vi "XY Graph Special Event Handler Core.vi"(8 "error in (no error)":errorcluster, 11 "XY Graph Event":T2) -> (0 "error out":errorcluster, 1 "Data":variant, 2 "Message":string, 3 "Menu Item Tag (dup)":string, 4 "Message Type":T1, 5 "Top Menu":string)   [LabVIEW 2021, in "XY Graph Add-Ons.lvlib"]
uses:
  XY Graph Add-Ons.lvlib
  XY Graph Event.ctl
  <vilib>/Utility/miscctls.llb/LVPoint32TypeDef.ctl
  Fits/Fit Plot Request Information.ctl
  <vilib>/Utility/miscctls.llb/LVPointDoubleTypeDef.ctl
  Fits/Fit Models.ctl
  XY Graph Mouse Click Event Data.ctl
  XY Graph Refnum.ctl
  XY Graph Save Plot Data.ctl
  Fits/Fits.lvlib
  Plot Editor/Plot Editor.lvlib
  Graphs.lvlib
  Histograms/Histogram Window.lvlib
  Strings/Strings.lvlib
  Rich Text Box/Text Format List.ctl
  Notebook/Notebook.lvlib
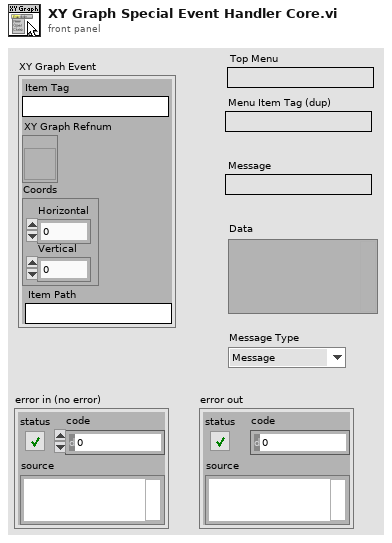
[diagram p1: front panel]
types:
  T1 = typedef "Notebook.lvlib/Text Format List.ctl" = enum16{"Message", "Result", "Error", "Setting", "Verbose", "Warning"}
  T2 = typedef "XY Graph Add-Ons.lvlib/XY Graph Event.ctl" = cluster{"Item Tag":string, "XY Graph Refnum":refnum<vi>, "Coords":T3, "Item Path":string}
  T3 = typedef "LVPoint32TypeDef.ctl" = cluster{"Horizontal":i32, "Vertical":i32}
  T4 = typedef "XY Graph Add-Ons.lvlib/XY Graph Mouse Click Event Data.ctl" = cluster{"Multiplot XY Graph":T5, "Mouse Coordinates":T3}
  T5 = typedef "XY Graph Add-Ons.lvlib/XY Graph Refnum.ctl" = refnum<vi>
  T6 = typedef "Fits.lvlib/Fit Plot Request Information.ctl" = cluster{"XY Graph Ref":refnum<vi>, "Mouse Coordinates":T7, "Fit Model":T8, "Plot Index":i32}
  T7 = typedef "LVPointDoubleTypeDef.ctl" = cluster{"X":dbl, "Y":dbl}
  T8 = typedef "Fits.lvlib/Fit Models.ctl" = enum16{"Select a Fit Model...", "           Single Peak", "Gaussian", "Asymmetric Gaussian", "Lorentzian", "Asymmetric Lorentzian", "Gaussian/Lorentzian", "Lorentzian/Gaussian", "           Double Peak", "Two Gaussians", "Two Asymmetric Gaussians", "Two H-Connected Gaussians", "Two T-Connected Gaussians", "Two H-Connected Asymmetric Gaussians", "Two T-Connected Asymmetric Gaussians", "           Triple Peak", "Three Gaussians", "Three Asymmetric Gaussians", "              Decays", "1-Exponential", "IRF*PSED", "2-Exponentials", "            Power Law", "Power Law", "Power Law with Offset", "               ACF", "2D Gaussian ACF", "2D Gaussian + Blinking ACF", "2D Gaussian + Flow ACF", "3D Gaussian ACF", "3D Gaussian + Blinking ACF", "             Multiplot", "2D Gaussian ACF & 2D Gaussian + Flow ACF"}
  T9 = typedef "XY Graph Add-Ons.lvlib/XY Graph Save Plot Data.ctl" = cluster{"XY Graph Refnum":refnum<vi>, "Mouse Coords":T3, "File Path":path}
  T10 = typedef "Graphs.lvlib/Plot Style 3.ctl" = cluster{"Plot Style":enum16{"unchanged", "Line", "Symbol", "Line + Symbol", "Histogram", "Histogram + Symbol"}, "Histogram Type":enum16{"unchanged", "Left Bound", "Center", "Right Bound"}, "Line Tickness":enum16{"unchanged", "Thin", "1 pixel", "2 pixel", "3 pixel", "4 pixel", "5 pixel"}, "Line Style":enum16{"unchanged", "Plain", "Long Dash", "Short Dash", "Long-Short Dash", "Long-Short-Short Dash"}, "Point Style":enum16{"unchanged", "None", "Empty Circle", "Filled Circle", "Thick Circle", "Dotted Circle", "Empty Square", "Filled Square", "Thick Square", "Dotted Square", "Small Filled Square", "Dot", "Cross", "Tiny Cross", "Large X", "Small x", "Diamond", "Small Empty Square"}, "Line Color":u32, "Point Color":u32, "Anti-aliased":bool, "Line Color Chooser":enum16{"unchanged", "Color Box", "Color List"}, "Point Color Chooser":enum16{"unchanged", "Color Box", "Color List"}, "Line Color List":string, "Point Color List":string}
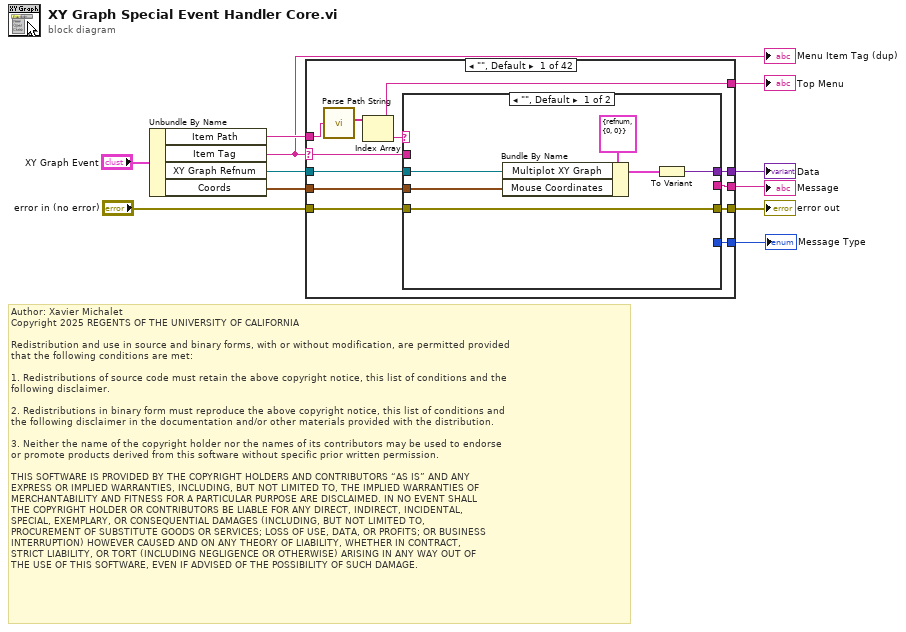
[diagram p0: block diagram]
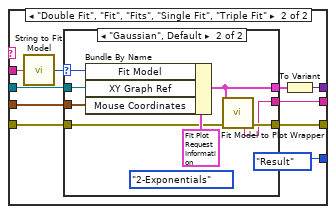
[diagram p2: hidden frame]
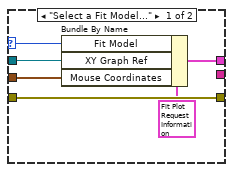
[diagram p3: hidden frame]
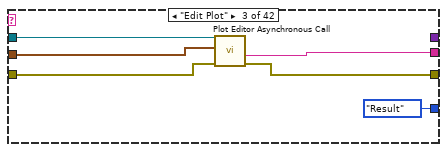
[diagram p5: hidden frame]
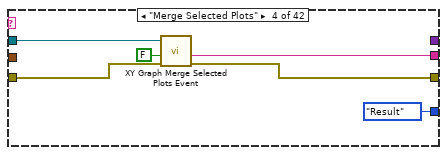
[diagram p6: hidden frame]
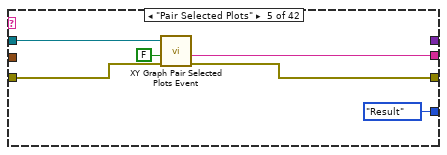
[diagram p7: hidden frame]
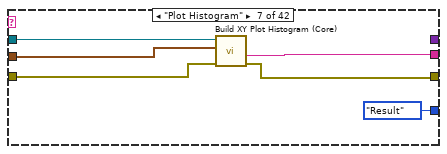
[diagram p9: hidden frame]
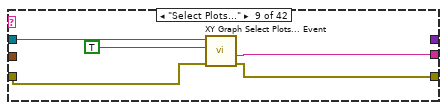
[diagram p11: hidden frame]
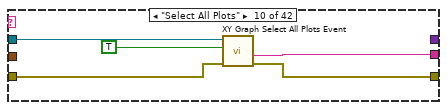
[diagram p12: hidden frame]
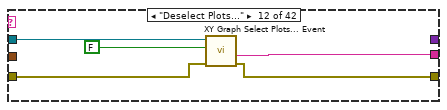
[diagram p14: hidden frame]
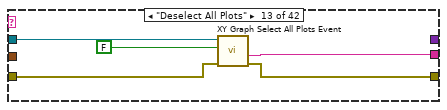
[diagram p15: hidden frame]
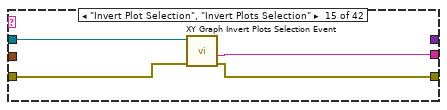
[diagram p17: hidden frame]
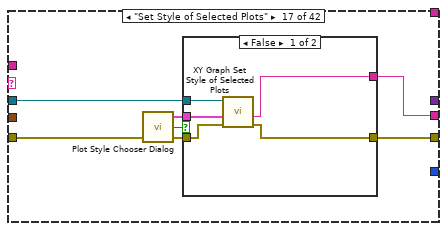
[diagram p19: hidden frame]
diagram:
  # "Author: Xavier Michalet\nCopyright 2025 REGENTS OF THE UNIVERSITY OF CALIFORNIA\n\nRedistribution and use in source and binary forms, with or without modification, are permitted provided\nthat the following conditions are met:\n\n1. Redistributions of source code must retain the above copyright notice, this list of conditions and the\nfollowing disclaimer.\n\n2. Redistributions in binary form must reproduce the above copyright notice, this list of conditions and\nthe following disclaimer in the documentation and/or other materials provided with the distribution.\n\n3. Neither the name of the copyright holder nor the names of its contributors may be used to endorse \nor promote products derived from this software without specific prior written permission.\n\nTHIS SOFTWARE IS PROVIDED BY THE COPYRIGHT HOLDERS AND CONTRIBUTORS “AS IS” AND ANY \nEXPRESS OR IMPLIED WARRANTIES, INCLUDING, BUT NOT LIMITED TO, THE IMPLIED WARRANTIES OF\nMERCHANTABILITY AND FITNESS FOR A PARTICULAR PURPOSE ARE DISCLAIMED. IN NO EVENT SHALL\nTHE COPYRIGHT HOLDER OR CONTRIBUTORS BE LIABLE FOR ANY DIRECT, INDIRECT, INCIDENTAL, \nSPECIAL, EXEMPLARY, OR CONSEQUENTIAL DAMAGES (INCLUDING, BUT NOT LIMITED TO, \nPROCUREMENT OF SUBSTITUTE GOODS OR SERVICES; LOSS OF USE, DATA, OR PROFITS; OR BUSINESS\nINTERRUPTION) HOWEVER CAUSED AND ON ANY THEORY OF LIABILITY, WHETHER IN CONTRACT, \nSTRICT LIABILITY, OR TORT (INCLUDING NEGLIGENCE OR OTHERWISE) ARISING IN ANY WAY OUT OF\nTHE USE OF THIS SOFTWARE, EVEN IF ADVISED OF THE POSSIBILITY OF SUCH DAMAGE."
  n1 = Unbundle By Name("XY Graph Event") -> ("Item Path"=w6:string, "Item Tag"=w5:string, "XY Graph Refnum"=w4:refnum<vi>, "Coords"=w3:T3)
  "Menu Item Tag (dup)" <- w5
  n2 = case shown="\"\", Default" w5 {
    selector: w5 -> [w20 _ _ _ _ _ _ _ _ _ _ _ _ _ _ _ _ _ _ _ _ _ _ _ _ _ _ _ _ _ _ _ _ _ _ _ _ _ _ _ _ _]
    tunnel: w4 -> [w22 _ w59 w65 w71 _ w78 _ w84 w89 _ w95 w100 _ w105 _ w110 w121 _ w131 w137 w141 _ w144 w153 w158 _ w167 w172 _ w180 _ w188 w194 _ w203 w211 w219 w224 _ w229 w233]
    tunnel: w3 -> [w21 _ w58 _ _ _ w77 _ _ _ _ _ _ _ _ _ _ _ _ w130 _ _ _ w143 _ _ _ _ _ _ w179 _ _ _ _ w202 w210 w218 _ _ _ _]
    tunnel: "error in (no error)" -> [w17 w53 w57 w63 w69 w72 w76 w79 w83 w87 w90 w94 w98 w101 w104 w106 w109 w123 w124 w129 w136 w140 w142 w149 w154 w159 w160 w166 w171 w173 w177 w182 w185 w191 w195 w200 w208 w216 w223 w225 w228 w232]
    tunnel: [w16 w53 w56 w62 w68 w72 w75 w79 w81 w85 w90 w92 w96 w101 w103 w106 w108 w122 w124 w127 w135 w139 w142 w148 w152 w157 w160 w165 w168 w173 w176 w182 w186 w192 w195 w199 w207 w215 w222 w225 w227 w231] -> w10
    tunnel: [w15 _ w55 w61 w67 _ w74 _ w80 w86 _ w91 w97 _ w102 _ w107 w120 _ w128 w134 w138 _ w147 w150 w155 _ w164 w170 _ w175 _ w184 w190 _ w198 w206 w214 w221 _ w226 w230] -> w11
    tunnel: w6 -> [w19 _ _ _ _ _ _ _ _ _ _ _ _ _ _ _ _ _ _ _ _ _ _ _ _ _ _ _ _ _ _ _ _ _ _ _ _ _ _ _ _ _]
    tunnel: [w14 _ _ _ _ _ _ _ _ _ _ _ _ _ _ _ _ _ _ w125 w132 _ _ _ _ _ _ w163 w169 _ _ _ _ _ _ _ _ _ _ _ _ _] -> w8
    tunnel: [w13 _ _ _ _ _ _ _ _ _ _ _ _ _ _ _ _ _ _ _ _ _ _ _ _ _ _ _ _ _ _ _ _ _ _ _ _ _ _ _ _ _] -> w2
    tunnel: [w12 _ Text_Format_List."Result" ("Message Type") Text_Format_List."Result" ("Message Type") Text_Format_List."Result" ("Message Type") _ Text_Format_List."Result" ("Message Type") _ _ _ _ _ _ _ _ _ _ _ _ _ _ _ _ _ _ _ _ _ _ _ Text_Format_List."Result" ("Message Type") _ Text_Format_List."Result" ("Message Type") Text_Format_List."Result" ("Message Type") _ Text_Format_List."Result" ("Message Type") Text_Format_List."Result" ("Message Type") Text_Format_List."Result" ("Message Type") Text_Format_List."Result" ("Message Type") _ _ _] -> w1
    frame "", Default {
      (unwired) T6 {"XY Graph Ref"=refnum, "Mouse Coordinates"={"X"=0.0, "Y"=0.0}, "Fit Model"=enum."Select a Fit Model...", "Plot Index"=-1} ("output cluster")
      n3 = call "Parse Path String.vi"("Path in"=w19) -> ("Folder Hierarchy"=w18:string[])  [unwired: 4 in, 1 out]
      n4 = Index Array(array=w18) -> (element=w13:string)  [unwired: 1 in]
      n5 = case shown="\"\", Default" w13 {
        tunnel: w22 -> [w26 w38]
        tunnel: w21 -> [w25 w37]
        tunnel: w20 -> [_ w36]
        tunnel: w17 -> [w28 w34]
        tunnel: [w28 w33] -> w16
        tunnel: [_ w32] -> w15
        tunnel: [w23 w30] -> w14
        tunnel: [_ Text_Format_List."Result" ("Message Type")] -> w12
        frame "", Default {
          n6 = Bundle By Name(cluster=T4 {"Multiplot XY Graph"=refnum, "Mouse Coordinates"={"Horizontal"=0, "Vertical"=0}} ("Mouse Click Event Data"), "Multiplot XY Graph"=w26, "Mouse Coordinates"=w25) -> (w24:T4)
          n7 = To Variant(anything=w24) -> (Variant=w23:variant)
        }
        frame "Double Fit", "Fit", "Fits", "Single Fit", "Triple Fit" {
          n8 = call "String to Fit Model.vi"("String"=w36) -> ("Fit Model"=w35:T8)  [unwired: 8 in]
          n9 = case shown="\"Gaussian\", Default" w35 {
            selector: w35 -> [w43 w49]
            tunnel: w38 -> [w42 w50]
            tunnel: w37 -> [w41 w51]
            tunnel: w34 -> [w44 w48]
            tunnel: [w44 w47] -> w33
            tunnel: [_ w46] -> w32
            tunnel: [w39 w45] -> w31
            frame "Select a Fit Model..." {
              n10 = Bundle By Name(cluster=T6 {"XY Graph Ref"=refnum, "Mouse Coordinates"={"X"=0.0, "Y"=0.0}, "Fit Model"=enum."Select a Fit Model...", "Plot Index"=0} ("Fit Plot Info"), "Fit Model"=w43, "XY Graph Ref"=w42, "Mouse Coordinates"=w41) -> (w39:T6)
            }
            frame "Gaussian", Default {
              (unwired) Fit_Models."2-Exponentials" ("Fit Model")
              n11 = Bundle By Name(cluster=T6 {"XY Graph Ref"=refnum, "Mouse Coordinates"={"X"=0.0, "Y"=0.0}, "Fit Model"=enum."Select a Fit Model...", "Plot Index"=-1} ("output cluster"), "Fit Model"=w49, "XY Graph Ref"=w50, "Mouse Coordinates"=w51) -> (w45:T6)
              n12 = call "Fit Model to Plot Wrapper.vi"("Fit Plot Info"=w45, "error in (no error)"=w48) -> ("Fit Result String"=w46:string, "error out"=w47:errorcluster)  [unwired: 5 in, 7 out]
            }
          }
          n13 = To Variant(anything=w31) -> (Variant=w30:variant)
        }
      }
    }
    frame "---------" {
    }
    frame "Edit Plot" {
      n14 = call "Plot Editor Asynchronous Call.vi"("error in (no error)"=w57, "Coords"=w58, "XYGraph in"=w59) -> ("Error Out"=w56:errorcluster, "Message"=w55:string)  [unwired: 5 in, 2 out]
    }
    frame "Merge Selected Plots" {
      n15 = call "XY Graph Merge Selected Plots Event.vi"("Error In"=w63, "Merge All Plots? (T)"=FALSE, "XY Graph Refnum"=w65) -> ("Error Out"=w62:errorcluster, "Message"=w61:string)  [unwired: 7 in]
    }
    frame "Pair Selected Plots" {
      n16 = call "XY Graph Pair Selected Plots Event.vi"("Error In"=w69, "Transpose?"=FALSE ("Merge All Plots? (T)"), "XYGraph Ref"=w71) -> ("Error Out"=w68:errorcluster, "Message"=w67:string)  [unwired: 7 in]
    }
    frame "-------------" {
    }
    frame "Plot Histogram" {
      n17 = call "Build XY Plot Histogram (Core).vi"("error in (no error)"=w76, "Mouse Click Coords (default: use Plot Index)"=w77, "XY Graph"=w78) -> ("error out"=w75:errorcluster, "Message"=w74:string)  [unwired: 6 in, 1 out]
    }
    frame "----------------" {
    }
    frame "Select Plots..." {
      n18 = call "XY Graph Select Plots... Event.vi"("Error In"=w83, "Select (T)/Deselect"=TRUE, "XYGraph Ref"=w84) -> ("Error Out"=w81:errorcluster, "Message"=w80:string)  [unwired: 4 in, 3 out]
    }
    frame "Select All Plots" {
      n19 = call "XY Graph Select All Plots Event.vi"("Error In"=w87, "Select (T)/Deselect"=TRUE, "XYGraph Ref"=w89) -> ("Error Out"=w85:errorcluster, "Message"=w86:string)  [unwired: 5 in, 2 out]
    }
    frame "----------------------" {
    }
    frame "Deselect Plots..." {
      n20 = call "XY Graph Select Plots... Event.vi"("Error In"=w94, "Select (T)/Deselect"=FALSE, "XYGraph Ref"=w95) -> ("Error Out"=w92:errorcluster, "Message"=w91:string)  [unwired: 4 in, 3 out]
    }
    frame "Deselect All Plots" {
      n21 = call "XY Graph Select All Plots Event.vi"("Error In"=w98, "Select (T)/Deselect"=FALSE, "XYGraph Ref"=w100) -> ("Error Out"=w96:errorcluster, "Message"=w97:string)  [unwired: 5 in, 2 out]
    }
    frame "-----------------------" {
    }
    frame "Invert Plot Selection", "Invert Plots Selection" {
      n22 = call "XY Graph Invert Plots Selection Event.vi"("Error In"=w104, "XYGraph Ref"=w105) -> ("Error Out"=w103:errorcluster, "Message"=w102:string)  [unwired: 6 in, 2 out]
    }
    frame "---------------" {
    }
    frame "Set Style of Selected Plots" {
      n23 = call "Plot Style Chooser Dialog.vi"("Error In"=w109) -> ("Plot Style out"=w113:T10, "Cancelled?"=w112:bool, "Error Out"=w111:errorcluster)  [unwired: 6 in]
      n24 = case shown="False" w112 {
        tunnel: w110 -> [w118 _]
        tunnel: w113 -> [w117 _]
        tunnel: w111 -> [w116 w119]
        tunnel: [w115 w119] -> w108
        tunnel: [w114 _] -> w107
        frame False {
          n25 = call "XY Graph Set Style of Selected Plots.vi"("Error In"=w116, "Plot Style"=w117, "XYGraph Ref"=w118) -> ("Error Out"=w115:errorcluster, "Message"=w114:string)  [unwired: 5 in, 2 out]
        }
        frame True {
        }
      }
    }
    frame "Set Axes of Selected Plots" {
      n26 = call "XY Graph Graph Axes Chooser Dialog.vi"("Error In"=w123, "XYGraph Ref"=w121) -> ("Error Out"=w122:errorcluster, "Message"=w120:string)  [unwired: 6 in, 2 out]
    }
    frame "-----------------" {
    }
    frame "Delete Plot" {
      n27 = call "XY Graph Delete Plot Event.vi"("Error In"=w129, "Mouse Click Coordinates"=w130, "XYGraph Ref"=w131) -> ("Error Out"=w127:errorcluster, "Message"=w128:string, "Deleted Plot Index"=w126:i32)  [unwired: 4 in, 2 out]
      n28 = To Variant(anything=w126) -> (Variant=w125:variant)
    }
    frame "Delete Selected Plots" {
      n29 = call "XY Graph Delete Selected Plots Event.vi"("Error In"=w136, "XYGraph Ref"=w137) -> ("Error Out"=w135:errorcluster, "Message"=w134:string, "Deleted Plot Indices"=w133:i32[])  [unwired: 5 in, 2 out]
      n30 = To Variant(anything=w133) -> (Variant=w132:variant)
    }
    frame "Clear Graph", "Delete All Plots" {
      n31 = call "XY Graph Clear Event.vi"("Error In"=w140, "XYGraph Ref"=w141) -> ("Error Out"=w139:errorcluster, "Message"=w138:string)  [unwired: 7 in, 1 out]
    }
    frame "------------------" {
    }
    frame "Save Plot" {
      n32 = Bundle By Name(cluster=T9 {"XY Graph Refnum"=refnum, "Mouse Coords"={"Horizontal"=0, "Vertical"=0}, "File Path"=path ""} ("AliGator Save Plot Data"), "XY Graph Refnum"=w144, "Mouse Coords"=w143) -> (w145:T9)
      n33 = call "XY Graph Save Plot Event.vi"("Error In"=w149, "AliGator Save Plot Data"=w145) -> ("Error Out"=w148:errorcluster, "Message"=w147:string)  [unwired: 4 in, 4 out]
    }
    frame "Save Selected Plots" {
      n34 = call "XY Graph Save Selected Plots Event.vi"("Error In"=w154, "Save All Plots? (T)"=FALSE, "XYGraph Ref"=w153) -> ("Error Out"=w152:errorcluster, "Message"=w150:string)  [unwired: 3 in, 4 out]
    }
    frame "Save All Plots" {
      n35 = call "XY Graph Save Selected Plots Event.vi"("Error In"=w159, "Save All Plots? (T)"=TRUE, "XYGraph Ref"=w158) -> ("Error Out"=w157:errorcluster, "Message"=w155:string)  [unwired: 3 in, 4 out]
    }
    frame "------------" {
    }
    frame "Load Plot(s)" {
      n36 = call "XY Graph Load Plot(s) Event.vi"("Error In"=w166, "XYGraph Ref"=w167) -> ("Error Out"=w165:errorcluster, "Message"=w164:string, "# Plots Added"=w162:i32[])  [unwired: 4 in, 3 out]
      n37 = Add Array Elements(numeric array=w162) -> (sum=w161:i32)
      n38 = To Variant(anything=w161) -> (Variant=w163:variant)
    }
    frame "Paste Plot(s) from Clipboard" {
      n39 = call "XY Graph Copy Plot(s) from Clipboard.vi"("error in (no error)"=w171, "XYGraph Ref"=w172) -> ("error out"=w168:errorcluster, "Message"=w170:string, "Number of Plots Added"=w169:i32)  [unwired: 7 in]
    }
    frame "--------------------------" {
    }
    frame "Transpose Plot" {
      n40 = Bundle(cluster=T4 {"Multiplot XY Graph"=refnum, "Mouse Coordinates"={"Horizontal"=0, "Vertical"=0}} ("Mouse Click Event Data"), "Multiplot XY Graph"=w180, "Mouse Coordinates"=w179) -> (w178:T4)
      n41 = call "XY Graph Transpose Plot Event.vi"("Error In"=w177, "Mouse Click Event Data"=w178) -> ("Error Out"=w176:errorcluster, "Message"=w175:string)  [unwired: 6 in, 2 out]
    }
    frame "--------------------" {
    }
    frame "Add Selected Plots" {
      n42 = call "XY Graph Sum Selected Plots Event.vi"("Error In"=w185, "Add All Plots? (F)"=FALSE, "XYGraph Ref"=w188) -> ("Error Out"=w186:errorcluster, "Message"=w184:string)  [unwired: 3 in, 4 out]
    }
    frame "Add All Plots" {
      n43 = call "XY Graph Sum Selected Plots Event.vi"("Error In"=w191, "Add All Plots? (F)"=TRUE, "XYGraph Ref"=w194) -> ("Error Out"=w192:errorcluster, "Message"=w190:string)  [unwired: 3 in, 4 out]
    }
    frame "---------------------" {
    }
    frame "Plot Arithmetic", "Single Plot Arithmetic", "y -> f(y) Transform", "y >> f(y) Transform" {
      n44 = Bundle(cluster=T4 {"Multiplot XY Graph"=refnum, "Mouse Coordinates"={"Horizontal"=0, "Vertical"=0}} ("Mouse Click Event Data"), "Multiplot XY Graph"=w203, "Mouse Coordinates"=w202) -> (w201:T4)
      n45 = call "XY Graph Compute Simple Plot Formula Event.vi"("Error In"=w200, "Mouse Click Event Data"=w201) -> ("Error Out"=w199:errorcluster, "Message"=w198:string)  [unwired: 5 in, 3 out]
    }
    frame "Interpolate Plot" {
      n46 = Bundle(cluster=T4 {"Multiplot XY Graph"=refnum, "Mouse Coordinates"={"Horizontal"=0, "Vertical"=0}} ("Mouse Click Event Data"), "Multiplot XY Graph"=w211, "Mouse Coordinates"=w210) -> (w209:T4)
      n47 = call "XY Graph Interpolate Plot Event.vi"("Error In"=w208, "Mouse Click Event Data"=w209) -> ("Error Out"=w207:errorcluster, "Message"=w206:string)  [unwired: 6 in, 2 out]
    }
    frame "(x, y) -> (f, g)(x, y) Transform", "(x, y) >> (f, g)(x, y) Transform", "Plot Transform", "Single Plot Transform" {
      n48 = Bundle(cluster=T4 {"Multiplot XY Graph"=refnum, "Mouse Coordinates"={"Horizontal"=0, "Vertical"=0}} ("Mouse Click Event Data"), "Multiplot XY Graph"=w219, "Mouse Coordinates"=w218) -> (w217:T4)
      n49 = call "XY Graph Compute Complex Plot Formula Event.vi"("Error In"=w216, "Mouse Click Event Data"=w217) -> ("Error Out"=w215:errorcluster, "Message"=w214:string)  [unwired: 5 in, 3 out]
    }
    frame "Multiplot Math" {
      n50 = call "XY Graph Compute Multiplot Math Event.vi"("Error In"=w223, "Multiplot XY Graph"=w224) -> ("Error Out"=w222:errorcluster, "Message"=w221:string)  [unwired: 6 in, 2 out]
    }
    frame "-------------------" {
    }
    frame "Grid", "Show/Hide Grid" {
      n51 = call "XY Graph Show-Hide Grid Event.vi"("Error In"=w228, "XYGraph Ref in"=w229) -> ("Error Out"=w227:errorcluster, "Message"=w226:string)  [unwired: 6 in, 2 out]
    }
    frame "Show/Hide Tool Panels", "Tool Panels" {
      n52 = call "XY Graph Show-Hide Tool Panels Event.vi"("Error In"=w232, "XYGraph in"=w233) -> ("Error Out"=w231:errorcluster, "Message"=w230:string)  [unwired: 7 in, 1 out]
    }
  }
  "Message" <- w11
  "error out" <- w10
  "Data" <- w8
  "Top Menu" <- w2
  "Message Type" <- w1
